vi "Main.vi"   [LabVIEW 2009]
types:
  T1 = enum32{"Invalid", "Standard", "Closed", "Hidden", "Minimized", "Maximized"}
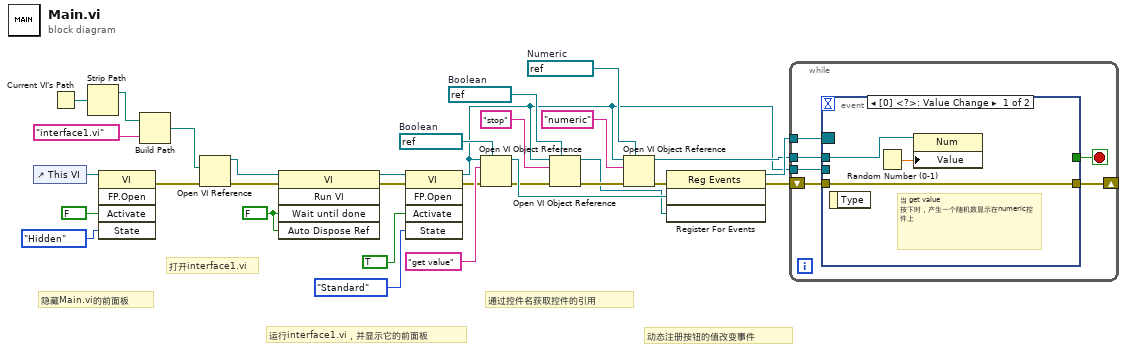
[diagram p0: block diagram]
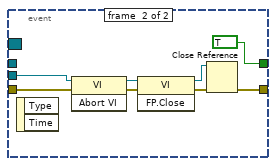
[diagram p2: hidden frame]
diagram:
  w8 = refnum<vi> refnum  # Numeric
  w11 = refnum<vi> refnum  # Boolean
  w15 = refnum<vi> refnum  # Boolean
  w26 = FALSE
  # "动态注册按钮的值改变事件"
  # "通过控件名获取控件的引用"
  # "运行interface1.vi，并显示它的前面板"
  # "打开interface1.vi"
  # "隐藏Main.vi的前面板"
  n1 = control-ref of="This VI"() -> (w24:refnum<vi>)
  n2 = Current VI's Path() -> (path=w31:path)
  n3 = Strip Path(path=w31) -> (stripped path=w30:path)  [unwired: 1 out]
  n4 = invoke class="VI" method="FP.Open"(reference=w24, "Activate"=FALSE ("Activate?"), "State"=T1."Hidden") -> (error out=w17:errorcluster)  [unwired: 2 in, 4 out]
  n5 = Build Path(base path=w30, name or relative path="interface1.vi" ("界面VI的名称")) -> (appended path=w28:path)
  n6 = Open VI Reference(vi path=w28, error in (no error)=w17) -> (vi reference=w27:refnum<vi>, error out=w25:errorcluster)  [unwired: 4 in]
  n7 = invoke class="VI" method="Run VI"(reference=w27, error in=w25, "Wait until done"=w26, "Auto Dispose Ref"=w26) -> (reference out=w21:refnum<vi>, error out=w20:errorcluster)  [unwired: 1 in, 3 out]
  n8 = invoke class="VI" method="FP.Open"(reference=w21, error in=w20, "Activate"=TRUE ("Activate?"), "State"=T1."Standard") -> (reference out=w2:refnum<vi>, error out=w13:errorcluster)  [unwired: 1 in, 3 out]
  n9 = Open VI Object Reference(7:w15, 8:w13, 10:"get value" ("name/order"), 11:w2) -> (0:w12:errorcluster, 3:w14:refnum<vi>)
  n10 = Open VI Object Reference(7:w11, 8:w12, 10:"stop" ("name/order"), 11:w2) -> (0:w7:errorcluster, 3:w6:refnum<vi>)
  n11 = Open VI Object Reference(7:w8, 8:w7, 10:"numeric" ("name/order"), 11:w2) -> (0:w4:errorcluster, 3:w3:refnum<vi>)
  n12 = register-events(error in=w4, w14, w6) -> (reference out=w5:refnum<event-registration>, error out=w1:errorcluster)  [unwired: 1 in]
  n13 = while {
    tunnel: w5 -> [w37]
    tunnel: w3 -> [w36]
    tunnel: w2 -> [w34]
    shift-right: [w32] -> _
    shift-left: w1 -> [w33]
    stop <- w35 stop-if-true
    n14 = event shown="[0] <?>: Value Change" {
      selector: w37 -> [_ _]
      dyn-events: _ -> [_ _]
      timeout: _ -> [_ _]
      tunnel: w36 -> [w40 _]
      tunnel: [_ TRUE] -> w35
      tunnel: w34 -> [_ w46]
      tunnel: w33 -> [w38 w45]
      tunnel: [w38 w47] -> w32
      event #0 {
        # "当 get value 按下时，产生一个随机数显示在numeric控件上"
        n15 = event-data() -> ()  [unwired: 1 in, 1 out]
        n16 = Random Number (0-1)() -> (number: 0 to 1=w39:dbl)
        n17 = property class="Num"(reference=w40, "Value"=w39) -> ()  [unwired: 1 in, 2 out]
      }
      event #1 {
        n18 = event-data() -> ()  [unwired: 1 in, 2 out]
        n19 = invoke class="VI" method="Abort VI"(reference=w46, error in=w45) -> (reference out=w44:refnum<vi>, error out=w43:errorcluster)  [unwired: 1 in, 1 out]
        n20 = invoke class="VI" method="FP.Close"(reference=w44, error in=w43) -> (reference out=w42:refnum<vi>, error out=w41:errorcluster)  [unwired: 1 in, 1 out]
        n21 = Close Reference(reference=w42, error in (no error)=w41) -> (error out=w47:errorcluster)
      }
    }
  }
